vi "PDC_GetMemFrameInfo.vi"(8 "error in (no error)":errorcluster, 10 "ChildNo":u32, 11 "DeviceNo":u32) -> (0 "error out":errorcluster, 2 "Frame":T1={"Start"=0, "End"=0, "Trigger"=0, "TwoStageLowToHigh"=0, "TwoStageHighToLow"=0, "TwoStageTiming"=0, "Event"=[1, 1, 1, 1, 1, 1, 1, 1, 1, 1], "EventCount"=0, "RecordedFrames"=0} {"RecordedFrames" max=0; "EventCount" max=0}, 3 "ReturnValue":u32, 4 "ErrorCode":u32)   [LabVIEW 2015]
doc: "This VI retrieves the frame information recorded in the current partition of the specified child device."
uses:
  PDCLIB.dll
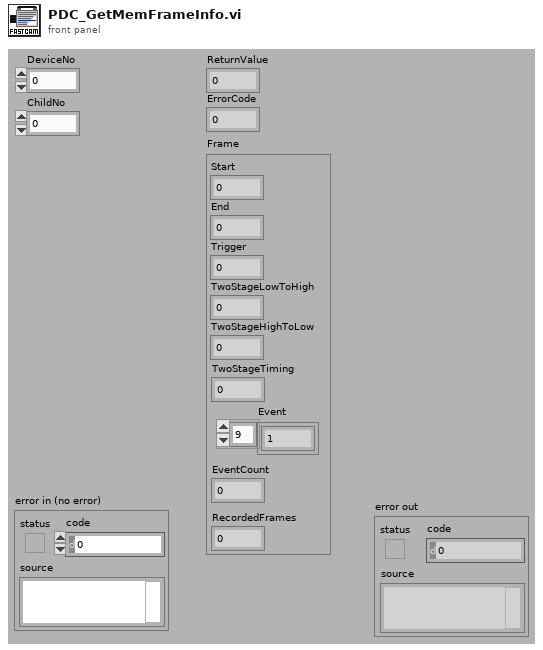
[diagram p1: front panel]
types:
  T1 = cluster{"Start":i32, "End":i32, "Trigger":i32, "TwoStageLowToHigh":i32, "TwoStageHighToLow":i32, "TwoStageTiming":u32, "Event":i32[], "EventCount":u32, "RecordedFrames":u32}
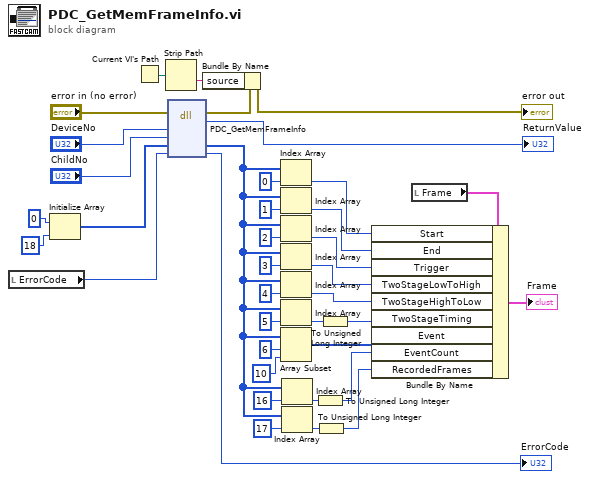
[diagram p0: block diagram]
diagram:
  n1 = local read "ErrorCode"() -> (w35:u32)
  n2 = Initialize Array(0 ("要素"), 18 ("次元サイズ")) -> (w26:i32[])
  n3 = Current VI's Path() -> (path=w31:path)
  n4 = Strip Path(path=w31) -> (name=w32:string)  [unwired: 1 out]
  n5 = dll-call lib="PDCLIB.dll" fn="PDC_GetMemFrameInfo"(error in="error in (no error)", "nDeviceNo"="DeviceNo", "nChildNo"="ChildNo", "pFrame"=w26, "pErrorCode"=w35) -> (error out=w30:errorcluster, "return type"=→"ReturnValue":u32, "pFrame"=w25:i32[], "pErrorCode"=→"ErrorCode":u32)  [unwired: 4 in, 1 out]
  n6 = Bundle By Name(cluster=w30, "source"=w32) -> (→"error out":errorcluster)
  n7 = Index Array(array=w25, index=0 ("指標")) -> (element=w12:i32)
  n8 = Index Array(array=w25, index=1 ("指標")) -> (element=w11:i32)
  n9 = Index Array(array=w25, index=2 ("指標")) -> (element=w10:i32)
  n10 = Index Array(array=w25, index=3 ("指標")) -> (element=w9:i32)
  n11 = Index Array(array=w25, index=4 ("指標")) -> (element=w8:i32)
  n12 = Index Array(array=w25, index=5 ("指標")) -> (element=w5:i32)
  n13 = Array Subset(array=w25, index=6 ("指標"), length=10 ("長さ")) -> (w7:i32[])
  n14 = Index Array(array=w25, index=16 ("指標")) -> (element=w3:i32)
  n15 = Index Array(array=w25, index=17 ("指標")) -> (element=w2:i32)
  n16 = To Unsigned Long Integer(number=w3) -> (unsigned 32bit integer=w4:u32)
  n17 = To Unsigned Long Integer(number=w2) -> (unsigned 32bit integer=w1:u32)
  n18 = To Unsigned Long Integer(number=w5) -> (unsigned 32bit integer=w6:u32)
  n19 = local read "Frame"() -> (w14:T1)
  n20 = Bundle By Name(cluster=w14, "Start"=w12, "End"=w11, "Trigger"=w10, "TwoStageLowToHigh"=w9, "TwoStageHighToLow"=w8, "TwoStageTiming"=w6, "Event"=w7, "EventCount"=w4, "RecordedFrames"=w1) -> (→"Frame":T1)
